vi "V_Measure_Score.vi"(8 "error in (no error)":errorcluster caption="entrée d'erreur (pas d'erreur)", 9 "labels_pred":string[][](array[string]), 10 "labels_true":string[][](array[string]), 11 "v_measure_score":cluster{"beta":dbl}={"beta"=1.0}) -> (0 "error out":errorcluster caption="sortie d'erreur", 3 "Score":string)   [LabVIEW 2020]
doc: "V-measure cluster labeling given a ground truth.\n\nThis score is identical to normalized_mutual_info_score with the 'arithmetic' option for averaging.\n\nThe V-measure is the harmonic mean between homogeneity and completeness:\n\nv = (1 + beta) * homogeneity * completeness\n / (beta * homogeneity + completeness)\nThis metric is independent of the absolute values of the labels: a permutation of the class or cluster label values won’t change the score value in any way.\n\nThis metric is furthermore symmetric: switching label_true with label_pred will return the same score value. This can be useful to measure the agreement of two independent label assignments strategies on the same dataset when the real ground truth is not known.\n\n\nParameters : \n\n- labels_true : int array, shape = [n_samples]\nground truth class labels to be used as a reference\n\n- labels_pred : array-like of shape (n_samples,)\ncluster labels to evaluate\n\n- beta : float\nRatio of weight attributed to homogeneity vs completeness. If beta is greater than 1, completeness is weighted more strongly in the calculation. If beta is less than 1, homogeneity is weighted more strongly.\n\nReturns : \n\n- v_measure : float\nscore between 0.0 and 1.0. 1.0 stands for perfectly complete labeling"
uses:
  V_Measure_Score.lvclass
panel:
  out "V_Measure_Score.lvclass":refnum<class "V_Measure_Score.lvclass">
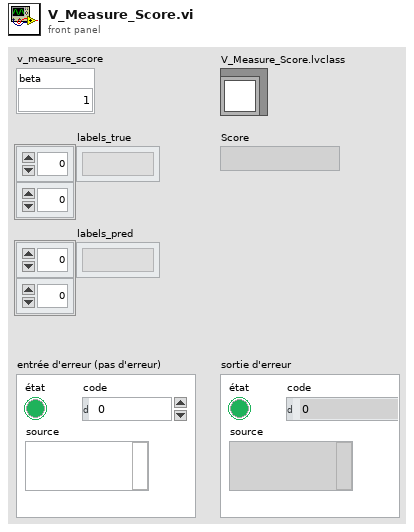
[diagram p1: front panel]
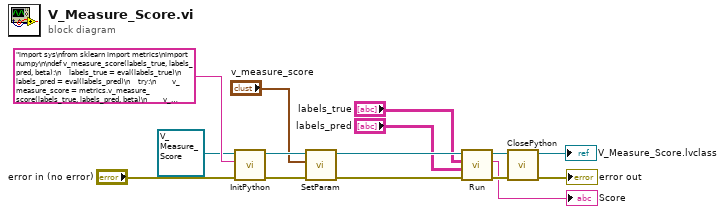
[diagram p0: block diagram]
diagram:
  n1 = call-dynamic "InitPython.vi"("error in (no error)"="error in (no error)", "Python Instruction"="import sys\nfrom sklearn import metrics\nimport numpy\n\ndef v_measure_score(labels_true, labels_pred, beta):\n    labels_true = eval(labels_true)\n    labels_pred = eval(labels_pred)\n    try:\n        v_measure_score = metrics.v_measure_score(labels_true, labels_pred, beta)\n        v_measure_score = v_measure_score.tolist()\n        return str(v_measure_score)\n    except:\n        erreur = sys.exc_info()\n        typerr = u\"%s\" % (erreur[0])\n        typerr = typerr[typerr.find(\"'\")+1:typerr.rfind(\"'\")]\n        msgerr = u\"%s\" % (erreur[1])\n        message = str('/!\\\\ {0} : {1}'. format(typerr,msgerr))\n        return message", "Scikit-learn en entrée"=refnum<class "V_Measure_Score.lvclass"> refnum ("V_Measure_Score.lvclass")) -> ("error out"=w11:errorcluster, "Scikit-learn en sortie"=w10:refnum<class "V_Measure_Score.lvclass">)  [unwired: 7 in]
  n2 = call-dynamic "SetParam.vi"("error in (no error)"=w11, "v_measure_score"="v_measure_score", "V_Measure_Score.lvclass"=w10) -> ("error out"=w7:errorcluster, "V_Measure_Score.lvclass"=w8:refnum<class "V_Measure_Score.lvclass">)  [unwired: 7 in]
  n3 = call-dynamic "Run.vi"("error in (no error)"=w7, "labels_pred"="labels_pred", "labels_true"="labels_true", "V_Measure_Score.lvclass"=w8) -> ("error out"=w6:errorcluster, "String Data"=→"Score":string, "V_Measure_Score.lvclass"=w5:refnum<class "V_Measure_Score.lvclass">)  [unwired: 5 in]
  n4 = call-dynamic "ClosePython.vi"("error in (no error)"=w6, "Scikit-learn en entrée"=w5) -> ("error out"=→"error out":errorcluster, "Scikit-learn en sortie"=→"V_Measure_Score.lvclass":refnum<class "V_Measure_Score.lvclass">)  [unwired: 8 in]
